vi "button_handler.vi"(7 "Disabled":T1(ring), 10 "reference":refnum<vi>[](array[refnum])) -> ()   [LabVIEW 2024]
doc: "This VI enables or disables or disables and greys-out all controls or indicators listed in the reference array input. It uses 2 inputs:\n- Disabled (required) : an Enum of 3 possible values (enables, disables or disables and greys-out)\n- reference : an Array of control or indicators references"
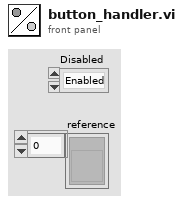
[diagram p1: front panel]
types:
  T1 = enum8{"Enabled", "Disabled", "Disabled and Grayed Out"}
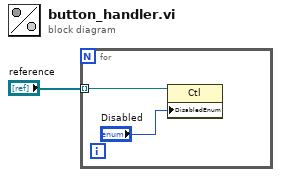
[diagram p0: block diagram]
diagram:
  n1 = for {
    tunnel: "reference" -> [w2] mode=indexing
    n2 = property class="Ctl"(reference=w2, "DisabledEnum"="Disabled") -> ()  [unwired: 1 in, 2 out]
  }
